vi "GetScanSpot.vi"(0 "Device to Scan":string) -> (1 "Scan Spot":string[](array[string]), 2 "Scanned Leads":string[](array[string]))   [LabVIEW 2015]
panel:
  out "Coordinates":dbl[][](array[numeric])
  in  "X edge odd":dbl=56.0
  in  "X edge even":dbl=-35.0
  in  "Y edge abcde":dbl=-73.0
  in  "Y edge efgh":dbl=-55.0
  # "Default scan corners for PCB Wafer lithography"
  # "All values here are cartesian coordinates"
  # "+y"
  # "Cartesian Coordinates"
  # "0,0"
  # "+x"
  # "-55"
  # "h\ng\nf\ne\nd\nc\nb\na"
  # "h\ng\nf\ne\nd\nc\nb\na"
  # "20x20\num"
  # "20x20\num"
  # "-75"
  # "-95"
  # "x="
  # "-35"
  # "-15"
  # "5"
  # "25"
  # "56"
  # "76"
  # "96"
  # "116"
  # "Decorations provide a scale depiction of 2x3 array of AFM images and their locations relative to the PCB lithographic crosshair.\nTop left corner is (x,y) for the leftmost AFM scan on any electrode.  After scanning at (x,y), the Auto-AFM routine scans again at (x+20,y) and (x+40,y).  Spacing is designed for a scan size = 21um, with a slight overlap of the 3 images and full coverage of the electrodes."
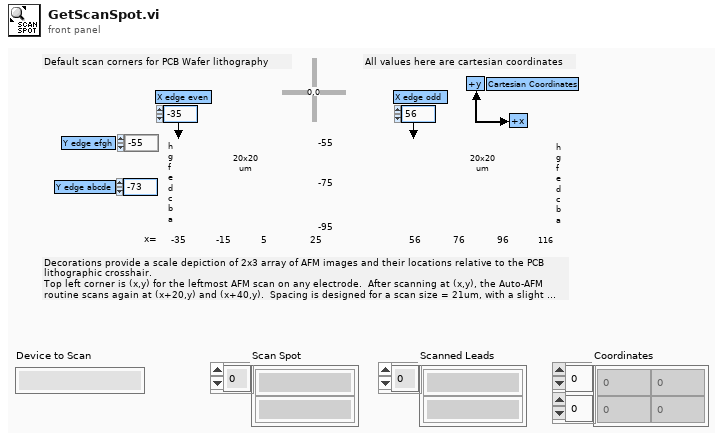
[diagram p1: front panel]
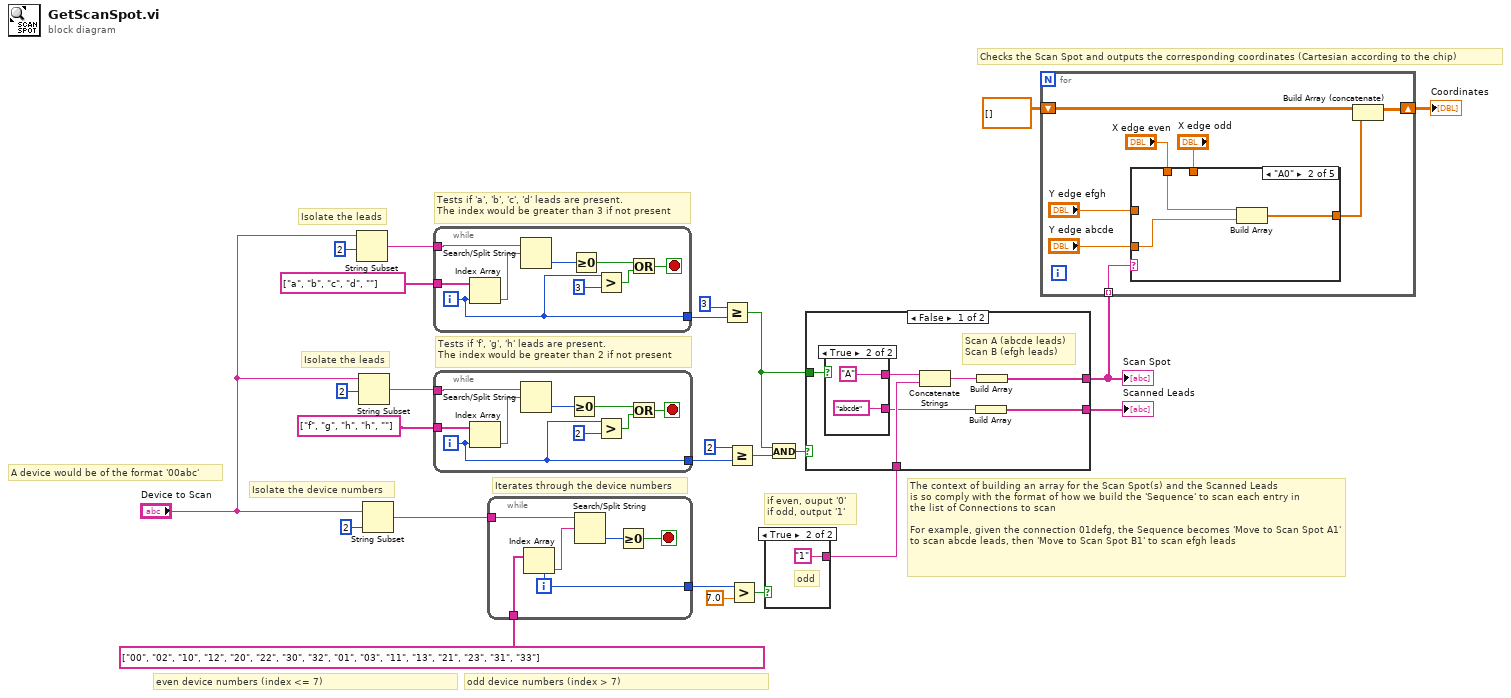
[diagram p0: block diagram]
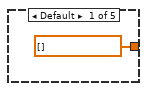
[diagram p2: hidden frame]
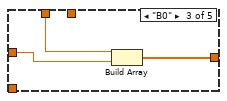
[diagram p3: hidden frame]
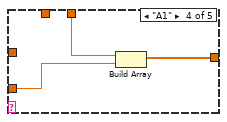
[diagram p4: hidden frame]
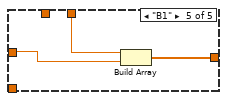
[diagram p5: hidden frame]
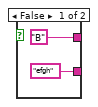
[diagram p6: hidden frame]
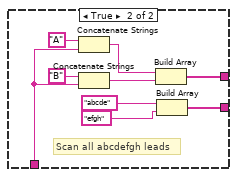
[diagram p7: hidden frame]
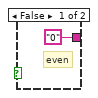
[diagram p8: hidden frame]
diagram:
  # "Checks the Scan Spot and outputs the corresponding coordinates (Cartesian according to the chip)"
  # "The context of building an array for the Scan Spot(s) and the Scanned Leads\nis so comply with the format of how we build the 'Sequence' to scan each entry in \nthe list of Connections to scan\n\nFor example, given the connection 01defg, the Sequence becomes 'Move to Scan Spot A1' to scan abcde leads, then 'Move to Scan Spot B1' to scan efgh leads"
  # "Isolate the device numbers"
  # "if even, ouput '0'\nif odd, output '1'"
  # "Iterates through the device numbers"
  # "odd device numbers (index > 7)"
  # "even device numbers (index <= 7)"
  # "Tests if 'f', 'g', 'h' leads are present. \nThe index would be greater than 2 if not present"
  # "Tests if 'a', 'b', 'c', 'd' leads are present. \nThe index would be greater than 3 if not present"
  # "Isolate the leads"
  # "Isolate the leads"
  # "A device would be of the format '00abc'"
  n1 = String Subset(string="Device to Scan", offset (0)=2 ("length (rest)")) -> (substring=w19:string)  [unwired: 1 in]
  n2 = String Subset(string="Device to Scan", offset (0)=2 ("length (rest)")) -> (substring=w17:string)  [unwired: 1 in]
  n3 = String Subset(string="Device to Scan", length (rest)=2 ("length (rest)")) -> (substring=w14:string)  [unwired: 1 in]
  n4 = while {
    tunnel: w19 -> [w32]
    tunnel: string[] ["a", "b", "c", "d", ""] -> [w34]
    tunnel: [w26] -> w9
    i -> [w26]
    stop <- w29 stop-if-true
    n5 = Index Array(array=w34, index=w26) -> (element=w33:string)
    n6 = Search/Split String(string=w32, search string/char (-)=w33) -> (offset of match=w31:i32)  [unwired: 1 in, 2 out]
    n7 = Greater Or Equal To 0?(x=w31) -> (x >= 0?=w30:bool)
    n8 = Greater?(x=w26, y=3) -> (0:w27:bool)
    n9 = Or(x=w30, y=w27) -> (x .or. y?=w29:bool)
  }
  n10 = while {
    tunnel: w17 -> [w41]
    tunnel: string[] ["f", "g", "h", "h", ""] -> [w43]
    tunnel: [w36] -> w7
    i -> [w36]
    stop <- w37 stop-if-true
    n11 = Index Array(array=w43, index=w36) -> (element=w42:string)
    n12 = Search/Split String(string=w41, search string/char (-)=w42) -> (offset of match=w40:i32)  [unwired: 1 in, 2 out]
    n13 = Greater Or Equal To 0?(x=w40) -> (x >= 0?=w38:bool)
    n14 = Greater?(x=w36, y=2) -> (0:w39:bool)
    n15 = Or(x=w38, y=w39) -> (x .or. y?=w37:bool)
  }
  n16 = while {
    tunnel: w14 -> [w48]
    tunnel: [w46] -> w11
    tunnel: string[] ["00", "02", "10", "12", "20", "22", "30", "32", "01", "03", "11", "13", "21", "23", "31", "33"] -> [w45]
    i -> [w46]
    stop <- w44 stop-if-true
    n17 = Index Array(array=w45, index=w46) -> (element=w49:string)
    n18 = Search/Split String(string=w48, search string/char (-)=w49) -> (offset of match=w47:i32)  [unwired: 1 in, 2 out]
    n19 = Greater Or Equal To 0?(x=w47) -> (x >= 0?=w44:bool)
  }
  n20 = Greater Or Equal?(x=3 ("y"), y=w9) -> (x >= y?=w12:bool)
  n21 = Greater Or Equal?(x=2 ("y"), y=w7) -> (x >= y?=w15:bool)
  n22 = Greater?(x=w11, y=7.0) -> (0:w23:bool)
  n23 = case shown="True" w23 {
    tunnel: ["0" "1"] -> w5
    frame False {
      # "even"
    }
    frame True {
      # "odd"
    }
  }
  n24 = And(x=w12, y=w15) -> (x .and. y?=w6:bool)
  n25 = case shown="False" w6 {
    tunnel: w12 -> [w58 _]
    tunnel: w5 -> [w57 w66]
    tunnel: [w54 w67] -> w3
    tunnel: [w53 w65] -> w4
    frame False {
      # "Scan A (abcde leads)\nScan B (efgh leads)"
      n26 = case shown="True" w58 {
        tunnel: ["B" "A"] -> w56
        tunnel: ["efgh" "abcde"] -> w52
        frame False {
        }
        frame True {
        }
      }
      n27 = Concatenate Strings(w56, w57) -> (w55:string)
      n28 = Build Array(w52) -> (w53:string[])
      n29 = Build Array(w55) -> (w54:string[])
    }
    frame True {
      # "Scan all abcdefgh leads"
      n30 = Concatenate Strings("A", w66) -> (w69:string)
      n31 = Concatenate Strings("B", w66) -> (w68:string)
      n32 = Build Array(w69, w68) -> (w67:string[])
      n33 = Build Array("abcde", "efgh") -> (w65:string[])
    }
  }
  "Scan Spot" <- w3
  "Scanned Leads" <- w4
  n34 = for {
    tunnel: w3 -> [w79] mode=indexing
    shift-right: [w73] -> w1
    shift-left: dbl[][] [] -> [w72]
    n35 = case shown="\"A0\"" w79 {
      tunnel: "X edge even" -> [_ w82 w86 _ _]
      tunnel: "X edge odd" -> [_ _ _ w89 w91]
      tunnel: "Y edge efgh" -> [_ _ w85 _ w90]
      tunnel: "Y edge abcde" -> [_ w83 _ w88 _]
      tunnel: [dbl[] [] w81 w84 w87 w92] -> w74
      frame Default {
      }
      frame "A0" {
        n36 = Build Array(w82, w83) -> (w81:dbl[])
      }
      frame "B0" {
        n37 = Build Array(w86, w85) -> (w84:dbl[])
      }
      frame "A1" {
        n38 = Build Array(w89, w88) -> (w87:dbl[])
      }
      frame "B1" {
        n39 = Build Array(w91, w90) -> (w92:dbl[])
      }
    }
    n40 = Build Array (concatenate)(w72, w74) -> (w73:dbl[][])
  }
  "Coordinates" <- w1
